vi "manage_accelero (SubVI).vi"(1 "Data in":T1) -> (8 "Data out":T1)   [LabVIEW 2015]
uses:
  data_typedef.ctl
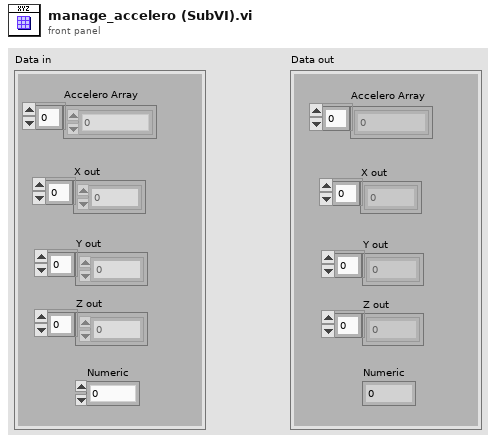
[diagram p1: front panel]
types:
  T1 = typedef "data_typedef.ctl" = cluster{"Accelero Array":dbl[], "Z out":dbl[], "Y out":dbl[], "X out":dbl[], "Numeric":i32}
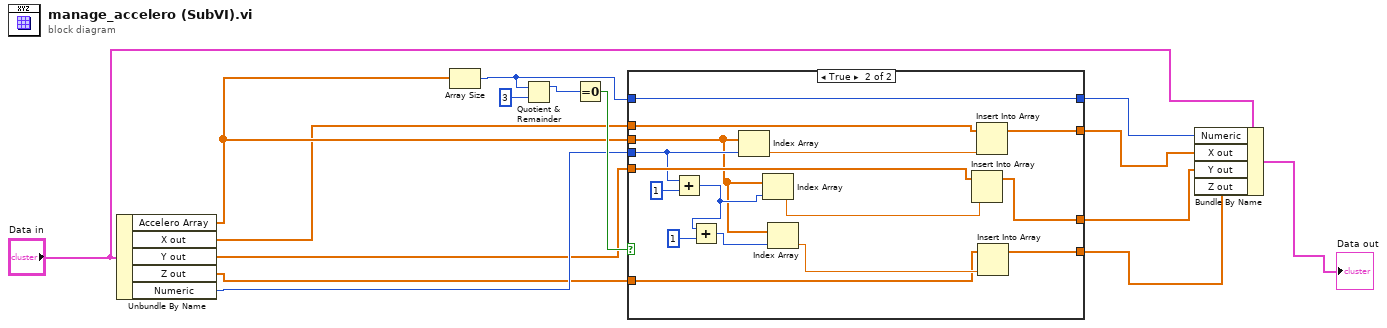
[diagram p0: block diagram]
diagram:
  n1 = Unbundle By Name("Data in") -> ("Accelero Array"=w12:dbl[], "X out"=w10:dbl[], "Y out"=w9:dbl[], "Z out"=w8:dbl[], "Numeric"=w11:i32)
  n2 = Array Size(array=w12) -> (size(s)=w3:i32)
  n3 = Quotient & Remainder(x=w3, y=3) -> (x-y*floor(x/y)=w13:i32)  [unwired: 1 out]
  n4 = Equal To 0?(x=w13) -> (x = 0?=w14:bool)
  n5 = case shown="True" w14 {
    tunnel: w10 -> [w19 w28]
    tunnel: w9 -> [w18 w27]
    tunnel: w8 -> [w17 w26]
    tunnel: [w17 w25] -> w4
    tunnel: [w18 w24] -> w5
    tunnel: [w19 w23] -> w6
    tunnel: w11 -> [w16 w22]
    tunnel: w12 -> [_ w21]
    tunnel: [w16 w20] -> w7
    tunnel: w3 -> [_ w20]
    frame False {
    }
    frame True {
      n6 = Add(x=w22, y=1) -> (x+y=w33:i32)
      n7 = Add(x=w33, y=1) -> (x+y=w32:i32)
      n8 = Index Array(array=w21, index=w22) -> (element=w31:dbl)
      n9 = Index Array(array=w21, index=w33) -> (element=w30:dbl)
      n10 = Index Array(array=w21, index=w32) -> (element=w29:dbl)
      n11 = Insert Into Array(array=w27, new element=w30) -> (w24:dbl[])  [unwired: 1 in]
      n12 = Insert Into Array(array=w28, new element=w31) -> (w23:dbl[])  [unwired: 1 in]
      n13 = Insert Into Array(array=w26, new element=w29) -> (w25:dbl[])  [unwired: 1 in]
    }
  }
  n14 = Bundle By Name(cluster="Data in", "Numeric"=w7, "X out"=w6, "Y out"=w5, "Z out"=w4) -> (→"Data out":T1)
